vi "Set Generic Property.vi"(0 "SLSC Local in":refnum<class "SLSC Local.lvclass">, 1 "property type":T1, 5 "resources":string, 7 "property":refnum<k21>, 9 "property value":variant, 11 "error in (no error)":errorcluster) -> (4 "SLSC Local out":refnum<class "SLSC Local.lvclass">, 15 "error out":errorcluster)   [LabVIEW 2015, in "SLSC Local.lvclass"]
uses:
  SLSC Local.lvclass
  SLSC Interface Class/Property Type.ctl
  <vilib>/SLSC/Set Device Property (DBL).vi
  <vilib>/SLSC/Set Device Property (I32).vi
  <vilib>/SLSC/Set Device Property (I64).vi
  <vilib>/SLSC/Set Device Property (U32).vi
  <vilib>/SLSC/Set Device Property (U64).vi
  <vilib>/SLSC/Set Device Property (1D Bool).vi
  <vilib>/SLSC/Set Device Property (1D DBL).vi
  <vilib>/SLSC/Set Device Property (1D I32).vi
  <vilib>/SLSC/Set Device Property (1D I64).vi
  <vilib>/SLSC/Set Device Property (1D String).vi
  <vilib>/SLSC/Set Device Property (1D U32).vi
  <vilib>/SLSC/Set Device Property (1D U64).vi
  <vilib>/SLSC/Set Generic Property (Bool).vi
  <vilib>/SLSC/Set Device Property (String).vi
  <vilib>/SLSC/SLSC.lvlib
  SLSC Interface Class/SLSC Interface.lvclass
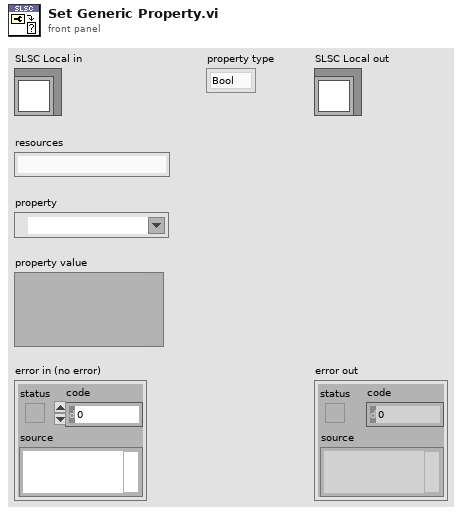
[diagram p1: front panel]
types:
  T1 = typedef "SLSC Interface.lvclass/Property Type.ctl" = enum16{"Bool", "DBL", "I32", "I64", "String", "U32", "U64", "1D Bool", "1D DBL", "1D I32", "1D I64", "1D String", "1D U32", "1D U64"}
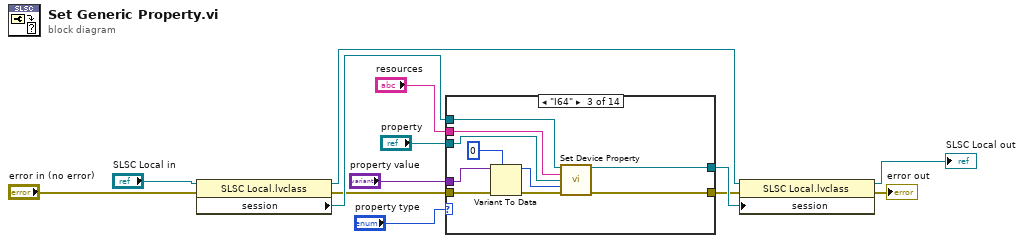
[diagram p0: block diagram]
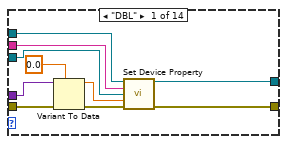
[diagram p2: hidden frame]
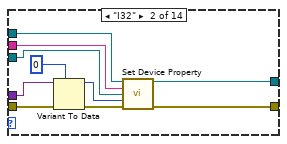
[diagram p3: hidden frame]
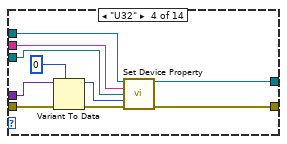
[diagram p4: hidden frame]
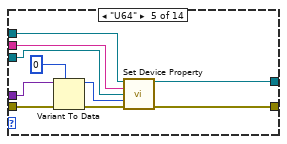
[diagram p5: hidden frame]
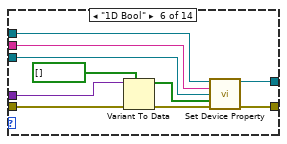
[diagram p6: hidden frame]
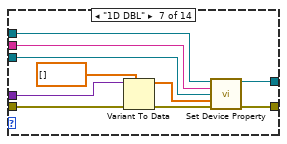
[diagram p7: hidden frame]
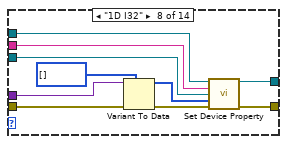
[diagram p8: hidden frame]
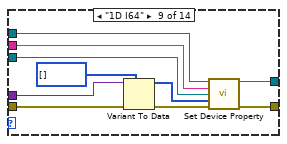
[diagram p9: hidden frame]
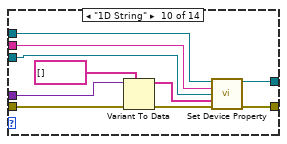
[diagram p10: hidden frame]
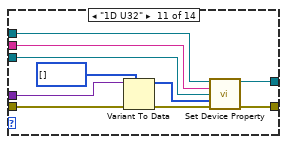
[diagram p11: hidden frame]
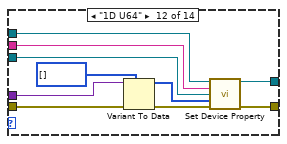
[diagram p12: hidden frame]
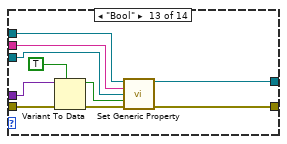
[diagram p13: hidden frame]
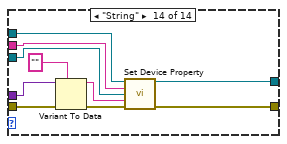
[diagram p14: hidden frame]
diagram:
  n1 = property class="SLSC Local.lvclass"(reference="SLSC Local in", error in="error in (no error)") -> (reference out=w6:refnum<class "SLSC Local.lvclass">, error out=w3:errorcluster, "session"=w8:refnum<k21>)
  n2 = case shown="\"I64\"" "property type" {
    tunnel: [w23 w33 w43 w53 w63 w73 w83 w93 w103 w113 w123 w133 w143 w153] -> w7
    tunnel: "resources" -> [w22 w32 w42 w52 w62 w72 w82 w92 w102 w112 w122 w132 w135 w152]
    tunnel: "property" -> [w21 w31 w41 w51 w61 w71 w81 w91 w101 w111 w121 w131 w142 w151]
    tunnel: w3 -> [w16 w26 w36 w46 w56 w66 w76 w86 w96 w106 w116 w126 w137 w146]
    tunnel: [w20 w30 w40 w50 w60 w70 w80 w90 w100 w110 w120 w130 w141 w150] -> w2
    tunnel: "property value" -> [w19 w29 w39 w49 w59 w69 w79 w89 w99 w109 w119 w129 w140 w149]
    tunnel: w8 -> [w14 w24 w34 w44 w54 w64 w74 w84 w94 w104 w114 w124 w134 w144]
    frame "DBL" {
      n3 = Variant To Data(error in=w16, type=0.0 ("property value"), Variant=w19) -> (data=w17:dbl, error out=w15:errorcluster)
      n4 = call-poly <vilib>:"Set Device Property.vi"("session in"=w14, "devices"=w22, "property"=w21, "property value"=w17, "error in (no error)"=w15) -> ("session out"=w23:refnum<k21>, "error out"=w20:errorcluster)  [unwired: 9 in]
    }
    frame "I32" {
      n5 = Variant To Data(error in=w26, type=0 ("property value"), Variant=w29) -> (data=w27:i32, error out=w25:errorcluster)
      n6 = call-poly <vilib>:"Set Device Property.vi"("session in"=w24, "devices"=w32, "property"=w31, "property value"=w27, "error in (no error)"=w25) -> ("session out"=w33:refnum<k21>, "error out"=w30:errorcluster)  [unwired: 9 in]
    }
    frame "I64" {
      n7 = Variant To Data(error in=w36, type=i64 0 ("property value"), Variant=w39) -> (data=w37:i64, error out=w35:errorcluster)
      n8 = call-poly <vilib>:"Set Device Property.vi"("session in"=w34, "devices"=w42, "property"=w41, "property value"=w37, "error in (no error)"=w35) -> ("session out"=w43:refnum<k21>, "error out"=w40:errorcluster)  [unwired: 9 in]
    }
    frame "U32" {
      n9 = Variant To Data(error in=w46, type=u32 0 ("property value"), Variant=w49) -> (data=w47:u32, error out=w45:errorcluster)
      n10 = call-poly <vilib>:"Set Device Property.vi"("session in"=w44, "devices"=w52, "property"=w51, "property value"=w47, "error in (no error)"=w45) -> ("session out"=w53:refnum<k21>, "error out"=w50:errorcluster)  [unwired: 9 in]
    }
    frame "U64" {
      n11 = Variant To Data(error in=w56, type=u64 0 ("property value"), Variant=w59) -> (data=w57:u64, error out=w55:errorcluster)
      n12 = call-poly <vilib>:"Set Device Property.vi"("session in"=w54, "devices"=w62, "property"=w61, "property value"=w57, "error in (no error)"=w55) -> ("session out"=w63:refnum<k21>, "error out"=w60:errorcluster)  [unwired: 9 in]
    }
    frame "1D Bool" {
      n13 = Variant To Data(error in=w66, type=bool[] [], Variant=w69) -> (data=w67:bool[], error out=w65:errorcluster)
      n14 = call-poly <vilib>:"Set Device Property.vi"("session in"=w64, "devices"=w72, "property"=w71, "property value"=w67, "error in (no error)"=w65) -> ("session out"=w73:refnum<k21>, "error out"=w70:errorcluster)  [unwired: 9 in]
    }
    frame "1D DBL" {
      n15 = Variant To Data(error in=w76, type=dbl[] [], Variant=w79) -> (data=w77:dbl[], error out=w75:errorcluster)
      n16 = call-poly <vilib>:"Set Device Property.vi"("session in"=w74, "devices"=w82, "property"=w81, "property value"=w77, "error in (no error)"=w75) -> ("session out"=w83:refnum<k21>, "error out"=w80:errorcluster)  [unwired: 9 in]
    }
    frame "1D I32" {
      n17 = Variant To Data(error in=w86, type=i32[] [], Variant=w89) -> (data=w87:i32[], error out=w85:errorcluster)
      n18 = call-poly <vilib>:"Set Device Property.vi"("session in"=w84, "devices"=w92, "property"=w91, "property value"=w87, "error in (no error)"=w85) -> ("session out"=w93:refnum<k21>, "error out"=w90:errorcluster)  [unwired: 9 in]
    }
    frame "1D I64" {
      n19 = Variant To Data(error in=w96, type=i64[] [], Variant=w99) -> (data=w97:i64[], error out=w95:errorcluster)
      n20 = call-poly <vilib>:"Set Device Property.vi"("session in"=w94, "devices"=w102, "property"=w101, "property value"=w97, "error in (no error)"=w95) -> ("session out"=w103:refnum<k21>, "error out"=w100:errorcluster)  [unwired: 9 in]
    }
    frame "1D String" {
      n21 = Variant To Data(error in=w106, type=string[] [], Variant=w109) -> (data=w107:string[], error out=w105:errorcluster)
      n22 = call-poly <vilib>:"Set Device Property.vi"("session in"=w104, "devices"=w112, "property"=w111, "property value"=w107, "error in (no error)"=w105) -> ("session out"=w113:refnum<k21>, "error out"=w110:errorcluster)  [unwired: 9 in]
    }
    frame "1D U32" {
      n23 = Variant To Data(error in=w116, type=u32[] [], Variant=w119) -> (data=w117:u32[], error out=w115:errorcluster)
      n24 = call-poly <vilib>:"Set Device Property.vi"("session in"=w114, "devices"=w122, "property"=w121, "property value"=w117, "error in (no error)"=w115) -> ("session out"=w123:refnum<k21>, "error out"=w120:errorcluster)  [unwired: 9 in]
    }
    frame "1D U64" {
      n25 = Variant To Data(error in=w126, type=u64[] [], Variant=w129) -> (data=w127:u64[], error out=w125:errorcluster)
      n26 = call-poly <vilib>:"Set Device Property.vi"("session in"=w124, "devices"=w132, "property"=w131, "property value"=w127, "error in (no error)"=w125) -> ("session out"=w133:refnum<k21>, "error out"=w130:errorcluster)  [unwired: 9 in]
    }
    frame "Bool" {
      n27 = Variant To Data(error in=w137, type=TRUE, Variant=w140) -> (data=w138:bool, error out=w136:errorcluster)
      n28 = call-poly <vilib>:"Set Generic Property.vi"("session in"=w134, "resources"=w135, "property"=w142, "property value"=w138, "error in (no error)"=w136) -> ("session out"=w143:refnum<k21>, "error out"=w141:errorcluster)  [unwired: 9 in]
    }
    frame "String" {
      n29 = Variant To Data(error in=w146, type="" ("property value"), Variant=w149) -> (data=w147:string, error out=w145:errorcluster)
      n30 = call-poly <vilib>:"Set Device Property.vi"("session in"=w144, "devices"=w152, "property"=w151, "property value"=w147, "error in (no error)"=w145) -> ("session out"=w153:refnum<k21>, "error out"=w150:errorcluster)  [unwired: 9 in]
    }
  }
  n31 = property class="SLSC Local.lvclass"(reference=w6, error in=w2, "session"=w7) -> (reference out=→"SLSC Local out":refnum<class "SLSC Local.lvclass">, error out=→"error out":errorcluster)
